vi "Get Status Pos.vi"(8 "error in (no error)":errorcluster caption="entrée d'erreur (pas d'erreur)", 11 "UI SA en entrée":refnum<class "UI SmarAct.lvclass">) -> (0 "error out":errorcluster caption="sortie d'erreur", 3 "UI SA en sortie":refnum<class "UI SmarAct.lvclass">)   [LabVIEW 2024, in "UI SmarAct.lvclass"]
uses:
  UI SmarAct.lvclass
  UI SmarAct.lvclass/UI SmarAct.ctl
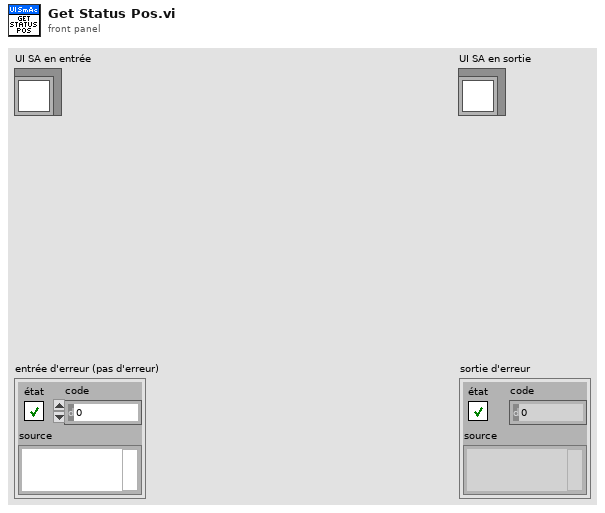
[diagram p1: front panel]
types:
  T1 = enum32{"SA_STOPPED_STATUS", "SA_STEPPING_STATUS", "SA_SCANNING_STATUS", "SA_HOLDING_STATUS", "SA_TARGET_STATUS", "SA_MOVE_DELAY_STATUS", "SA_CALIBRATING_STATUS", "SA_FINDING_REF_STATUS", "SA_OPENING_STATUS"}
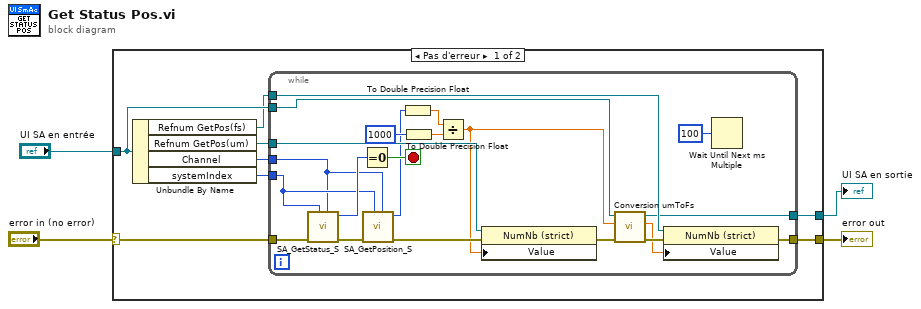
[diagram p0: block diagram]
diagram:
  n1 = case shown="Pas d'erreur" "error in (no error)" {
    selector: "error in (no error)" -> [w12 w35]
    tunnel: [w11 w35] -> w3
    tunnel: [w6 w34] -> w1
    tunnel: "UI SA en entrée" -> [w7 w34]
    frame No Error {
      n2 = Unbundle By Name(w7) -> ("Refnum GetPos(fs)"=w5:refnum<vi>, "Refnum GetPos(um)"=w8:refnum<vi>, "Channel"=w9:u32, "systemIndex"=w10:u32)
      n3 = while {
        tunnel: w12 -> [w32]
        tunnel: [w26] -> w11
        tunnel: w10 -> [w29]
        tunnel: w9 -> [w28]
        tunnel: w8 -> [w25]
        tunnel: w5 -> [w24]
        tunnel: w7 -> [w15]
        tunnel: [w14] -> w6
        stop <- w30 stop-if-true
        n4 = call <vilib>:"SA_GetStatus_S.vi"("channelIndex"=w28, "systemIndex"=w29, "error in (no error)"=w32) -> ("error out"=w33:errorcluster, "status"=w31:T1)  [unwired: 7 in]
        n5 = Equal To 0?(x=w31) -> (x = 0?=w30:bool)
        n6 = call <vilib>:"SA_GetPosition_S.vi"("channelIndex"=w28, "systemIndex"=w29, "error in (no error)"=w33) -> ("error out"=w27:errorcluster, "position"=w20:i32)  [unwired: 7 in]
        n7 = To Double Precision Float(number=w20) -> (double precision float=w23:dbl)
        n8 = To Double Precision Float(number=1000 ("y")) -> (double precision float=w22:dbl)
        n9 = Divide(x=w23, y=w22) -> (x/y=w16:dbl)
        n10 = property class="NumNb (strict)"(reference=w25, error in=w27, "Value"=w16) -> (error out=w19:errorcluster)  [unwired: 1 out]
        n11 = call "Conversion umToFs.vi"("error in (no error)"=w19, "um"=w16, "UI SA en entrée"=w15) -> ("error out"=w18:errorcluster, "Fs"=w17:ext, "UI SA en sortie"=w14:refnum<class "UI SmarAct.lvclass">)  [unwired: 6 in]
        n12 = property class="NumNb (strict)"(reference=w24, error in=w18, "Value"=w17) -> (error out=w26:errorcluster)  [unwired: 1 out]
        n13 = Wait Until Next ms Multiple(millisecond multiple=u32 100 ("n millisecondes")) -> ()  [unwired: 1 out]
      }
    }
    frame Error {
    }
  }
  "error out" <- w3
  "UI SA en sortie" <- w1
